vi "AT Set Float A.vi"(8 "error in (no error)":errorcluster, 9 "Value":dbl, 10 "Feature":string, 11 "Hndl":i32) -> (0 "error out":errorcluster, 3 "function return":i32)   [LabVIEW 2019]
doc: "Set float\n\nOutput:\n I32 Status\n\nInput:\n I32 Handle\n String Feature\n Double Value\n\nThis function will modify the value of the specified feature, if the feature is of float type. The function will return an error if the feature is read only or currently not writable or if the feature is either not a float type feature or is not implemented by the camera."
uses:
  atcoreA.dll
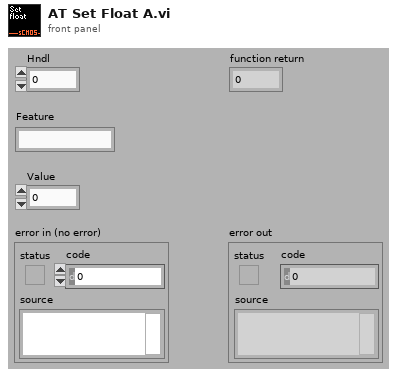
[diagram p1: front panel]
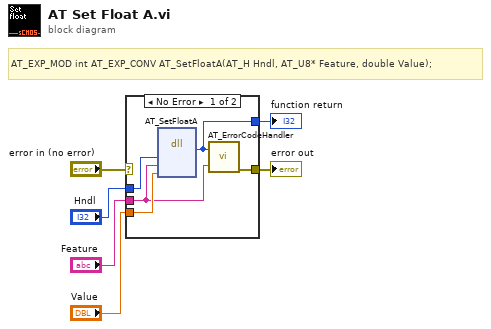
[diagram p0: block diagram]
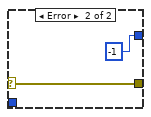
[diagram p2: hidden frame]
diagram:
  # "AT_EXP_MOD int AT_EXP_CONV AT_SetFloatA(AT_H Hndl, AT_U8* Feature, double Value);"
  n1 = case shown="No Error" "error in (no error)" {
    selector: "error in (no error)" -> [_ w13]
    tunnel: [w8 -1 ("return type")] -> w6
    tunnel: "Hndl" -> [w11 _]
    tunnel: "Feature" -> [w7 _]
    tunnel: "Value" -> [w10 _]
    tunnel: [w9 w13] -> w2
    frame No Error {
      n2 = dll-call lib="atcoreA.dll" fn="AT_SetFloatA"("Handle"=w11, "Feature"=w7, "Value"=w10) -> ("Status"=w8:i32)  [unwired: 6 in, 2 out]
      n3 = call <userlib>:"AT_ErrorCodeHandler.vi"("Error"=w8, "Feature Name"=w7) -> ("error out"=w9:errorcluster)  [unwired: 5 in]
    }
    frame Error {
    }
  }
  "function return" <- w6
  "error out" <- w2
